vi "Read both gates.vi"(8 "error in (no error)":errorcluster, 11 "VISA resource name":refnum<visa-resource-name>) -> (0 "Gate B Delay":dbl[unit] format="%^#_6g", 1 "Gate A Delay":dbl[unit] format="%^#_6g", 2 "Gate B Width":dbl[unit] format="%^#_6g", 3 "Gate A Width":dbl[unit] format="%^#_6g", 4 "Current mode B":enum16{"CW", "Fixed", "Scan"}(ring), 5 "Current mode A":enum16{"CW", "Fixed", "Scan"}(ring), 6 "error out":errorcluster, 7 "VISA resource name out":refnum<visa-resource-name>)   [LabVIEW 2015, in "SR400.lvlib"]
uses:
  SR400.lvlib
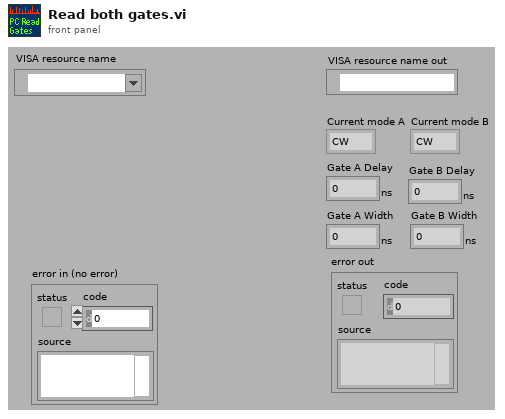
[diagram p1: front panel]
types:
  T1 = typedef "SR400.lvlib/Gate Mode.ctl" = enum16{"CW", "Fixed", "Scan"}
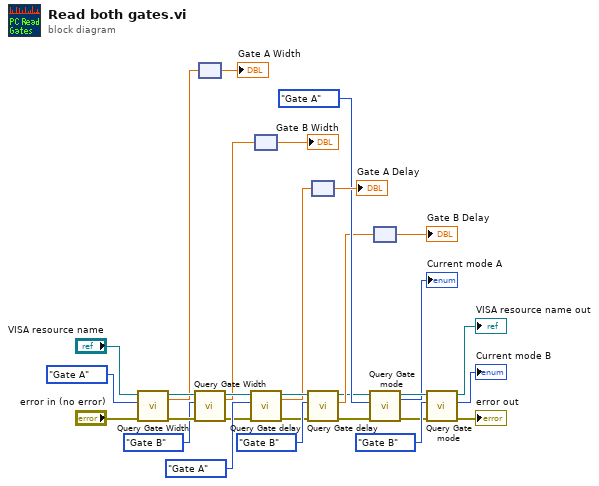
[diagram p0: block diagram]
diagram:
  n1 = call "Query Gate Width.vi"("error in (no error)"="error in (no error)", "Gate (def: A)"=enum16{"Gate A", "Gate B"}."Gate A" ("i (0)"), "VISA resource name"="VISA resource name") -> ("error out"=w9:errorcluster, "width (s)"=w4:dbl, "VISA resource name out"=w10:refnum<visa-resource-name>)  [unwired: 6 out]
  n2 = call "Query Gate Width.vi"("error in (no error)"=w9, "Gate (def: A)"=enum16{"Gate A", "Gate B"}."Gate B" ("i (0)"), "VISA resource name"=w10) -> ("error out"=w12:errorcluster, "width (s)"=w3:dbl, "VISA resource name out"=w11:refnum<visa-resource-name>)  [unwired: 6 out]
  n3 = node(w4) -> (→"Gate A Width":dbl[unit])
  n4 = call "Query Gate delay.vi"("error in (no error)"=w12, "Gate (def: A)"=enum16{"Gate A", "Gate B"}."Gate A" ("i (0)"), "VISA resource name"=w11) -> ("error out"=w15:errorcluster, "output"=w16:dbl, "VISA resource name out"=w20:refnum<visa-resource-name>)  [unwired: 6 out]
  n5 = node(w3) -> (→"Gate B Width":dbl[unit])
  n6 = call "Query Gate delay.vi"("error in (no error)"=w15, "Gate (def: A)"=enum16{"Gate A", "Gate B"}."Gate B" ("i (0)"), "VISA resource name"=w20) -> ("error out"=w14:errorcluster, "output"=w17:dbl, "VISA resource name out"=w13:refnum<visa-resource-name>)  [unwired: 6 out]
  n7 = node(w16) -> (→"Gate A Delay":dbl[unit])
  n8 = call "Query Gate mode.vi"("error in (no error)"=w14, "i (0)"=enum16{"Gate A", "Gate B"}."Gate A", "VISA resource name"=w13) -> ("error out"=w24:errorcluster, "Gate mode"=→"Current mode A":T1, "VISA resource name out"=w18:refnum<visa-resource-name>)  [unwired: 6 out]
  n9 = node(w17) -> (→"Gate B Delay":dbl[unit])
  n10 = call "Query Gate mode.vi"("error in (no error)"=w24, "i (0)"=enum16{"Gate A", "Gate B"}."Gate B", "VISA resource name"=w18) -> ("error out"=→"error out":errorcluster, "Gate mode"=→"Current mode B":T1, "VISA resource name out"=→"VISA resource name out":refnum<visa-resource-name>)  [unwired: 6 out]
